vi "square.vi"() -> ()   [LabVIEW 2025]
panel:
  out "square root":i32
  out "cube of  number":i32
  out "square of a num":i32
  in  "Enter a number":dbl
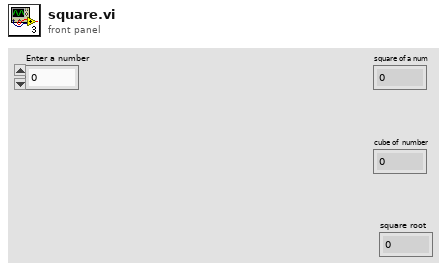
[diagram p1: front panel]
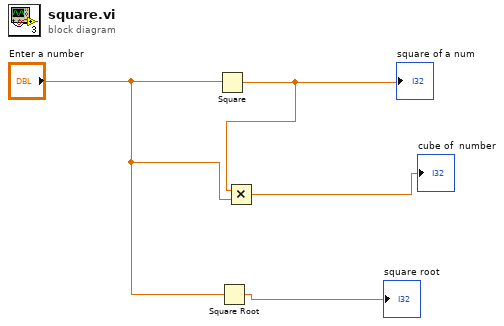
[diagram p0: block diagram]
diagram:
  n1 = Square(x="Enter a number") -> (x^2=w4:dbl)
  "square of a num" <- w4
  n2 = Square Root(x="Enter a number") -> (sqrt(x)=→"square root":dbl)
  n3 = Multiply(x=w4, y="Enter a number") -> (x*y=→"cube of  number":dbl)
